vi "matrice_led.vi"() -> ()   [LabVIEW 2018]
panel:
  out "temp":u32
  in  "stop":bool
  in  "Meter":u32(knob) scale=0.0..10.0
  in  "Combo Box":string(combo)
  out "LED1 32":bool
  out "LED1 31":bool
  out "LED1 30":bool
  out "LED1 29":bool
  out "LED1 28":bool
  out "LED1 27":bool
  out "LED1 26":bool
  out "LED1 25":bool
  out "LED1 24":bool
  out "LED1 23":bool
  out "LED1 22":bool
  out "LED1 21":bool
  out "LED1 20":bool
  out "LED1 19":bool
  out "LED1 18":bool
  out "LED1 17":bool
  out "LED1 16":bool
  out "LED1 15":bool
  out "LED1 14":bool
  out "LED1 13":bool
  out "LED1 12":bool
  out "LED1 11":bool
  out "LED1 10":bool
  out "LED1 9":bool
  out "LED1 8":bool
  out "LED1 7":bool
  out "LED1 6":bool
  out "LED1 5":bool
  out "LED1 4":bool
  out "LED1 3":bool
  out "LED1 2":bool
  out "LED1":bool
  # "SIMULAREA UNOR EFECTE GRAFICE VARIATE CARE POT FI AFISATE PE MATRICEA VIRTUALA DE 8X4 LEDURI"
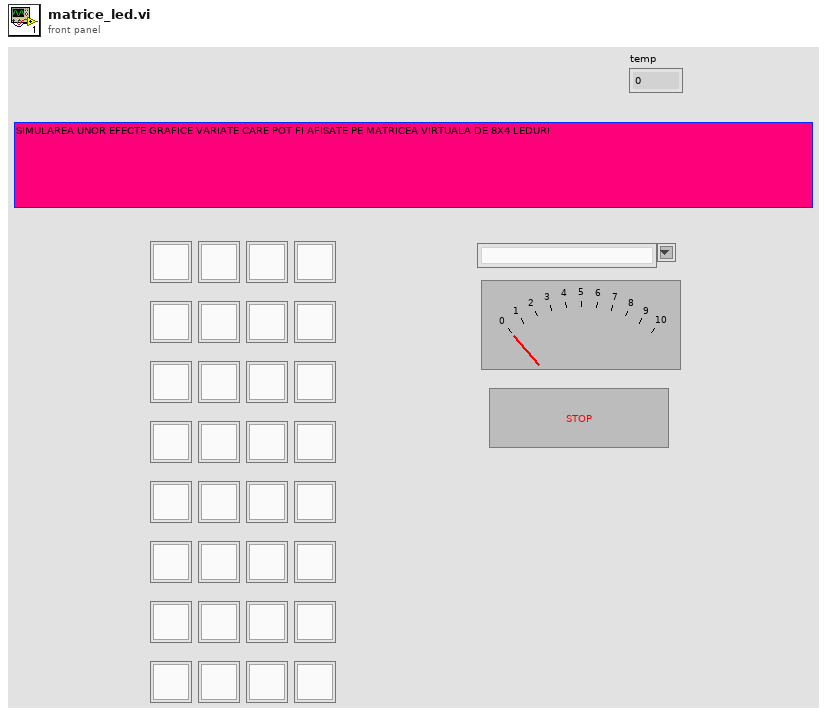
[diagram p1: front panel]
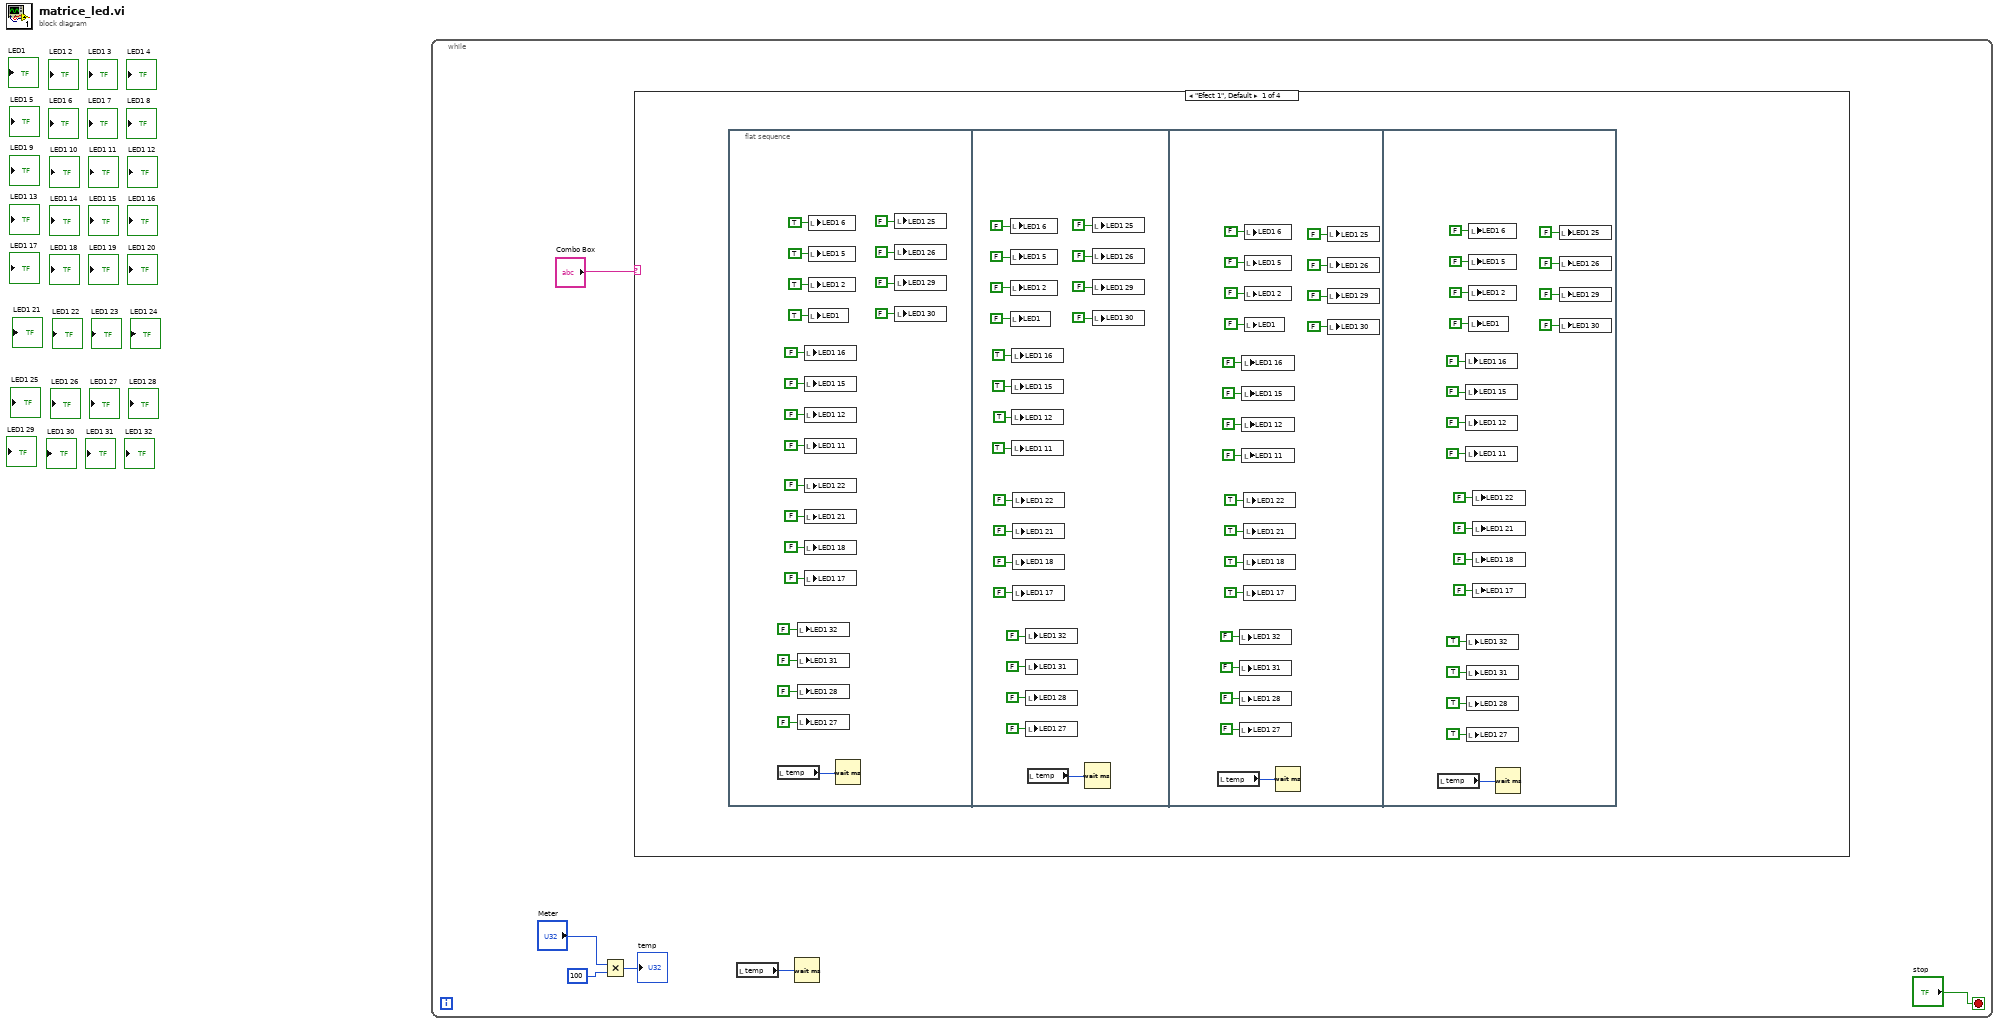
[diagram p0: block diagram]
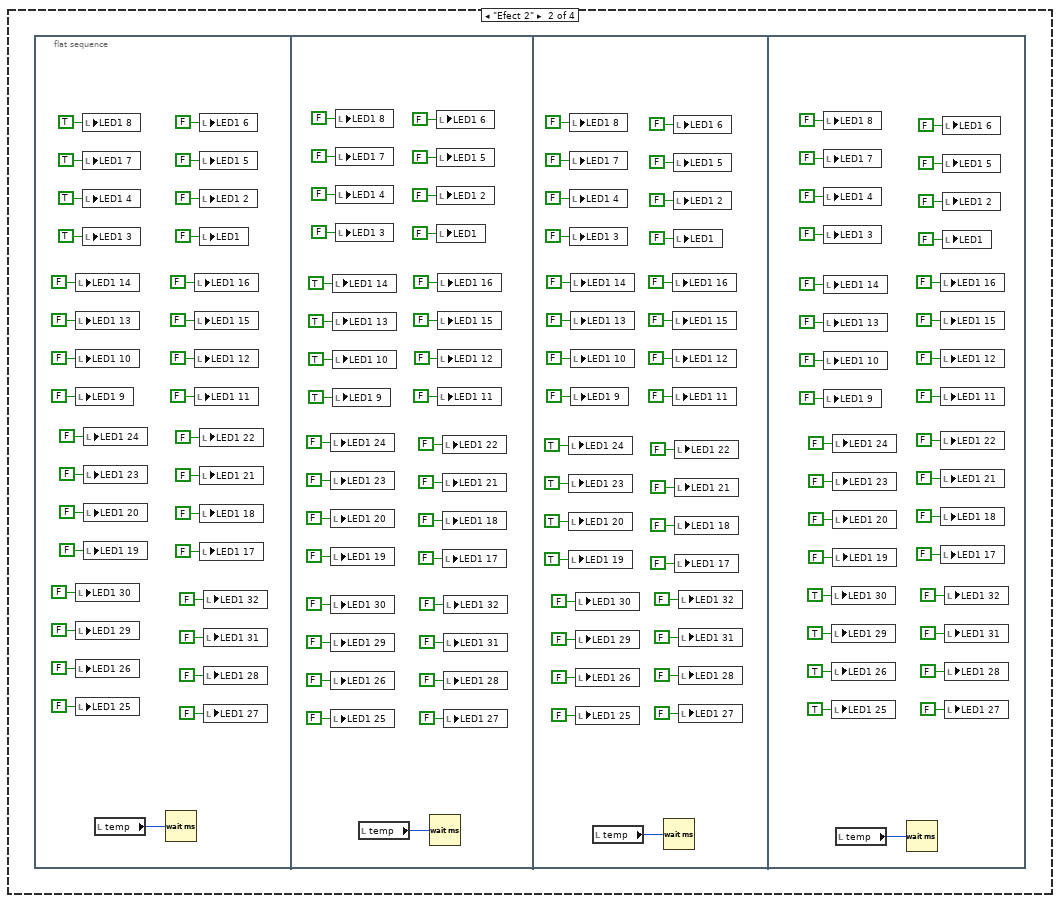
[diagram p2: hidden frame]
diagram:
  n1 = while {
    stop <- "stop" stop-if-true
    n2 = Multiply(x="Meter", y=u32 100) -> (x*y=→"temp":u32)
    n3 = case shown="\"Efect 1\", Default" "Combo Box" {
      frame "Efect 1", Default {
        n4 = flat-sequence {
          frame #0 {
            n5 = local read "temp"() -> (w27:u32)
            n6 = local write "LED1 32"(FALSE ("LED1 32")) -> ()
            n7 = local write "LED1 31"(FALSE ("LED1 31")) -> ()
            n8 = local write "LED1 28"(FALSE ("LED1 28")) -> ()
            n9 = local write "LED1 27"(FALSE ("LED1 27")) -> ()
            n10 = local write "LED1 16"(FALSE ("LED1 16")) -> ()
            n11 = local write "LED1 15"(FALSE ("LED1 15")) -> ()
            n12 = local write "LED1 12"(FALSE ("LED1 12")) -> ()
            n13 = local write "LED1 11"(FALSE ("LED1 11")) -> ()
            n14 = local write "LED1 22"(FALSE ("LED1 22")) -> ()
            n15 = local write "LED1 21"(FALSE ("LED1 21")) -> ()
            n16 = local write "LED1 18"(FALSE ("LED1 18")) -> ()
            n17 = local write "LED1 17"(FALSE ("LED1 17")) -> ()
            n18 = local write "LED1 6"(TRUE ("LED1 6")) -> ()
            n19 = local write "LED1 5"(TRUE ("LED1 5")) -> ()
            n20 = local write "LED1 2"(TRUE ("LED1 2")) -> ()
            n21 = local write "LED1"(TRUE ("LED1")) -> ()
            n22 = Wait (ms)(milliseconds to wait=w27) -> ()  [unwired: 1 out]
            n23 = local write "LED1 25"(FALSE ("LED1 25")) -> ()
            n24 = local write "LED1 26"(FALSE ("LED1 26")) -> ()
            n25 = local write "LED1 29"(FALSE ("LED1 29")) -> ()
            n26 = local write "LED1 30"(FALSE ("LED1 30")) -> ()
          }
          frame #1 {
            n27 = local write "LED1 6"(FALSE ("LED1 6")) -> ()
            n28 = local write "LED1 5"(FALSE ("LED1 5")) -> ()
            n29 = local write "LED1 2"(FALSE ("LED1 2")) -> ()
            n30 = local write "LED1"(FALSE ("LED1")) -> ()
            n31 = local write "LED1 16"(TRUE ("LED1 16")) -> ()
            n32 = local write "LED1 15"(TRUE ("LED1 15")) -> ()
            n33 = local write "LED1 12"(TRUE ("LED1 12")) -> ()
            n34 = local write "LED1 11"(TRUE ("LED1 11")) -> ()
            n35 = local write "LED1 22"(FALSE ("LED1 22")) -> ()
            n36 = local write "LED1 21"(FALSE ("LED1 21")) -> ()
            n37 = local write "LED1 18"(FALSE ("LED1 18")) -> ()
            n38 = local write "LED1 17"(FALSE ("LED1 17")) -> ()
            n39 = local write "LED1 32"(FALSE ("LED1 32")) -> ()
            n40 = local write "LED1 31"(FALSE ("LED1 31")) -> ()
            n41 = local write "LED1 28"(FALSE ("LED1 28")) -> ()
            n42 = local write "LED1 27"(FALSE ("LED1 27")) -> ()
            n43 = local read "temp"() -> (w48:u32)
            n44 = Wait (ms)(milliseconds to wait=w48) -> ()  [unwired: 1 out]
            n45 = local write "LED1 25"(FALSE ("LED1 25")) -> ()
            n46 = local write "LED1 26"(FALSE ("LED1 26")) -> ()
            n47 = local write "LED1 29"(FALSE ("LED1 29")) -> ()
            n48 = local write "LED1 30"(FALSE ("LED1 30")) -> ()
          }
          frame #2 {
            n49 = local read "temp"() -> (w69:u32)
            n50 = local write "LED1 32"(FALSE ("LED1 32")) -> ()
            n51 = local write "LED1 31"(FALSE ("LED1 31")) -> ()
            n52 = local write "LED1 28"(FALSE ("LED1 28")) -> ()
            n53 = local write "LED1 27"(FALSE ("LED1 27")) -> ()
            n54 = local write "LED1 16"(FALSE ("LED1 16")) -> ()
            n55 = local write "LED1 15"(FALSE ("LED1 15")) -> ()
            n56 = local write "LED1 12"(FALSE ("LED1 12")) -> ()
            n57 = local write "LED1 11"(FALSE ("LED1 11")) -> ()
            n58 = local write "LED1 22"(TRUE ("LED1 22")) -> ()
            n59 = local write "LED1 21"(TRUE ("LED1 21")) -> ()
            n60 = local write "LED1 18"(TRUE ("LED1 18")) -> ()
            n61 = local write "LED1 17"(TRUE ("LED1 17")) -> ()
            n62 = local write "LED1 6"(FALSE ("LED1 6")) -> ()
            n63 = local write "LED1 5"(FALSE ("LED1 5")) -> ()
            n64 = local write "LED1 2"(FALSE ("LED1 2")) -> ()
            n65 = local write "LED1"(FALSE ("LED1")) -> ()
            n66 = Wait (ms)(milliseconds to wait=w69) -> ()  [unwired: 1 out]
            n67 = local write "LED1 25"(FALSE ("LED1 25")) -> ()
            n68 = local write "LED1 26"(FALSE ("LED1 26")) -> ()
            n69 = local write "LED1 29"(FALSE ("LED1 29")) -> ()
            n70 = local write "LED1 30"(FALSE ("LED1 30")) -> ()
          }
          frame #3 {
            n71 = local read "temp"() -> (w90:u32)
            n72 = local write "LED1 16"(FALSE ("LED1 16")) -> ()
            n73 = local write "LED1 15"(FALSE ("LED1 15")) -> ()
            n74 = local write "LED1 12"(FALSE ("LED1 12")) -> ()
            n75 = local write "LED1 11"(FALSE ("LED1 11")) -> ()
            n76 = local write "LED1 32"(TRUE ("LED1 32")) -> ()
            n77 = local write "LED1 31"(TRUE ("LED1 31")) -> ()
            n78 = local write "LED1 28"(TRUE ("LED1 28")) -> ()
            n79 = local write "LED1 27"(TRUE ("LED1 27")) -> ()
            n80 = local write "LED1 6"(FALSE ("LED1 6")) -> ()
            n81 = local write "LED1 5"(FALSE ("LED1 5")) -> ()
            n82 = local write "LED1 2"(FALSE ("LED1 2")) -> ()
            n83 = local write "LED1"(FALSE ("LED1")) -> ()
            n84 = local write "LED1 22"(FALSE ("LED1 22")) -> ()
            n85 = local write "LED1 21"(FALSE ("LED1 21")) -> ()
            n86 = local write "LED1 18"(FALSE ("LED1 18")) -> ()
            n87 = local write "LED1 17"(FALSE ("LED1 17")) -> ()
            n88 = Wait (ms)(milliseconds to wait=w90) -> ()  [unwired: 1 out]
            n89 = local write "LED1 25"(FALSE ("LED1 25")) -> ()
            n90 = local write "LED1 26"(FALSE ("LED1 26")) -> ()
            n91 = local write "LED1 29"(FALSE ("LED1 29")) -> ()
            n92 = local write "LED1 30"(FALSE ("LED1 30")) -> ()
          }
        }
      }
      frame "Efect 2" {
        n93 = flat-sequence {
          frame #0 {
            n94 = local write "LED1 14"(FALSE ("LED1 14")) -> ()
            n95 = local write "LED1 13"(FALSE ("LED1 13")) -> ()
            n96 = local write "LED1 10"(FALSE ("LED1 10")) -> ()
            n97 = local write "LED1 9"(FALSE ("LED1 9")) -> ()
            n98 = local write "LED1 30"(FALSE ("LED1 30")) -> ()
            n99 = local write "LED1 29"(FALSE ("LED1 29")) -> ()
            n100 = local write "LED1 26"(FALSE ("LED1 26")) -> ()
            n101 = local write "LED1 25"(FALSE ("LED1 25")) -> ()
            n102 = local write "LED1 8"(TRUE ("LED1 8")) -> ()
            n103 = local write "LED1 7"(TRUE ("LED1 7")) -> ()
            n104 = local write "LED1 4"(TRUE ("LED1 4")) -> ()
            n105 = local write "LED1 3"(TRUE ("LED1 3")) -> ()
            n106 = local write "LED1 24"(FALSE ("LED1 24")) -> ()
            n107 = local write "LED1 23"(FALSE ("LED1 23")) -> ()
            n108 = local write "LED1 20"(FALSE ("LED1 20")) -> ()
            n109 = local write "LED1 19"(FALSE ("LED1 19")) -> ()
            n110 = local read "temp"() -> (w123:u32)
            n111 = Wait (ms)(milliseconds to wait=w123) -> ()  [unwired: 1 out]
            n112 = local write "LED1 16"(FALSE ("LED1 16")) -> ()
            n113 = local write "LED1 15"(FALSE ("LED1 15")) -> ()
            n114 = local write "LED1 12"(FALSE ("LED1 12")) -> ()
            n115 = local write "LED1 11"(FALSE ("LED1 11")) -> ()
            n116 = local write "LED1 6"(FALSE ("LED1 6")) -> ()
            n117 = local write "LED1 5"(FALSE ("LED1 5")) -> ()
            n118 = local write "LED1 2"(FALSE ("LED1 2")) -> ()
            n119 = local write "LED1"(FALSE ("LED1")) -> ()
            n120 = local write "LED1 22"(FALSE ("LED1 22")) -> ()
            n121 = local write "LED1 21"(FALSE ("LED1 21")) -> ()
            n122 = local write "LED1 18"(FALSE ("LED1 18")) -> ()
            n123 = local write "LED1 17"(FALSE ("LED1 17")) -> ()
            n124 = local write "LED1 32"(FALSE ("LED1 32")) -> ()
            n125 = local write "LED1 31"(FALSE ("LED1 31")) -> ()
            n126 = local write "LED1 28"(FALSE ("LED1 28")) -> ()
            n127 = local write "LED1 27"(FALSE ("LED1 27")) -> ()
          }
          frame #1 {
            n128 = local write "LED1 24"(FALSE ("LED1 24")) -> ()
            n129 = local write "LED1 23"(FALSE ("LED1 23")) -> ()
            n130 = local write "LED1 20"(FALSE ("LED1 20")) -> ()
            n131 = local write "LED1 19"(FALSE ("LED1 19")) -> ()
            n132 = local write "LED1 30"(FALSE ("LED1 30")) -> ()
            n133 = local write "LED1 29"(FALSE ("LED1 29")) -> ()
            n134 = local write "LED1 26"(FALSE ("LED1 26")) -> ()
            n135 = local write "LED1 25"(FALSE ("LED1 25")) -> ()
            n136 = local write "LED1 14"(TRUE ("LED1 14")) -> ()
            n137 = local write "LED1 13"(TRUE ("LED1 13")) -> ()
            n138 = local write "LED1 10"(TRUE ("LED1 10")) -> ()
            n139 = local write "LED1 9"(TRUE ("LED1 9")) -> ()
            n140 = local write "LED1 8"(FALSE ("LED1 8")) -> ()
            n141 = local write "LED1 7"(FALSE ("LED1 7")) -> ()
            n142 = local write "LED1 4"(FALSE ("LED1 4")) -> ()
            n143 = local write "LED1 3"(FALSE ("LED1 3")) -> ()
            n144 = local read "temp"() -> (w156:u32)
            n145 = Wait (ms)(milliseconds to wait=w156) -> ()  [unwired: 1 out]
            n146 = local write "LED1 6"(FALSE ("LED1 6")) -> ()
            n147 = local write "LED1 5"(FALSE ("LED1 5")) -> ()
            n148 = local write "LED1 2"(FALSE ("LED1 2")) -> ()
            n149 = local write "LED1"(FALSE ("LED1")) -> ()
            n150 = local write "LED1 16"(FALSE ("LED1 16")) -> ()
            n151 = local write "LED1 15"(FALSE ("LED1 15")) -> ()
            n152 = local write "LED1 12"(FALSE ("LED1 12")) -> ()
            n153 = local write "LED1 11"(FALSE ("LED1 11")) -> ()
            n154 = local write "LED1 22"(FALSE ("LED1 22")) -> ()
            n155 = local write "LED1 21"(FALSE ("LED1 21")) -> ()
            n156 = local write "LED1 18"(FALSE ("LED1 18")) -> ()
            n157 = local write "LED1 17"(FALSE ("LED1 17")) -> ()
            n158 = local write "LED1 32"(FALSE ("LED1 32")) -> ()
            n159 = local write "LED1 31"(FALSE ("LED1 31")) -> ()
            n160 = local write "LED1 28"(FALSE ("LED1 28")) -> ()
            n161 = local write "LED1 27"(FALSE ("LED1 27")) -> ()
          }
          frame #2 {
            n162 = local write "LED1 24"(TRUE ("LED1 24")) -> ()
            n163 = local write "LED1 23"(TRUE ("LED1 23")) -> ()
            n164 = local write "LED1 20"(TRUE ("LED1 20")) -> ()
            n165 = local write "LED1 19"(TRUE ("LED1 19")) -> ()
            n166 = local write "LED1 8"(FALSE ("LED1 8")) -> ()
            n167 = local write "LED1 7"(FALSE ("LED1 7")) -> ()
            n168 = local write "LED1 4"(FALSE ("LED1 4")) -> ()
            n169 = local write "LED1 3"(FALSE ("LED1 3")) -> ()
            n170 = local write "LED1 14"(FALSE ("LED1 14")) -> ()
            n171 = local write "LED1 13"(FALSE ("LED1 13")) -> ()
            n172 = local write "LED1 10"(FALSE ("LED1 10")) -> ()
            n173 = local write "LED1 9"(FALSE ("LED1 9")) -> ()
            n174 = local write "LED1 30"(FALSE ("LED1 30")) -> ()
            n175 = local write "LED1 29"(FALSE ("LED1 29")) -> ()
            n176 = local write "LED1 26"(FALSE ("LED1 26")) -> ()
            n177 = local write "LED1 25"(FALSE ("LED1 25")) -> ()
            n178 = local read "temp"() -> (w189:u32)
            n179 = Wait (ms)(milliseconds to wait=w189) -> ()  [unwired: 1 out]
            n180 = local write "LED1 16"(FALSE ("LED1 16")) -> ()
            n181 = local write "LED1 15"(FALSE ("LED1 15")) -> ()
            n182 = local write "LED1 12"(FALSE ("LED1 12")) -> ()
            n183 = local write "LED1 11"(FALSE ("LED1 11")) -> ()
            n184 = local write "LED1 6"(FALSE ("LED1 6")) -> ()
            n185 = local write "LED1 5"(FALSE ("LED1 5")) -> ()
            n186 = local write "LED1 2"(FALSE ("LED1 2")) -> ()
            n187 = local write "LED1"(FALSE ("LED1")) -> ()
            n188 = local write "LED1 22"(FALSE ("LED1 22")) -> ()
            n189 = local write "LED1 21"(FALSE ("LED1 21")) -> ()
            n190 = local write "LED1 18"(FALSE ("LED1 18")) -> ()
            n191 = local write "LED1 17"(FALSE ("LED1 17")) -> ()
            n192 = local write "LED1 32"(FALSE ("LED1 32")) -> ()
            n193 = local write "LED1 31"(FALSE ("LED1 31")) -> ()
            n194 = local write "LED1 28"(FALSE ("LED1 28")) -> ()
            n195 = local write "LED1 27"(FALSE ("LED1 27")) -> ()
          }
          frame #3 {
            n196 = local write "LED1 8"(FALSE ("LED1 8")) -> ()
            n197 = local write "LED1 7"(FALSE ("LED1 7")) -> ()
            n198 = local write "LED1 4"(FALSE ("LED1 4")) -> ()
            n199 = local write "LED1 3"(FALSE ("LED1 3")) -> ()
            n200 = local write "LED1 14"(FALSE ("LED1 14")) -> ()
            n201 = local write "LED1 13"(FALSE ("LED1 13")) -> ()
            n202 = local write "LED1 10"(FALSE ("LED1 10")) -> ()
            n203 = local write "LED1 9"(FALSE ("LED1 9")) -> ()
            n204 = local write "LED1 30"(TRUE ("LED1 30")) -> ()
            n205 = local write "LED1 29"(TRUE ("LED1 29")) -> ()
            n206 = local write "LED1 26"(TRUE ("LED1 26")) -> ()
            n207 = local write "LED1 25"(TRUE ("LED1 25")) -> ()
            n208 = local write "LED1 24"(FALSE ("LED1 24")) -> ()
            n209 = local write "LED1 23"(FALSE ("LED1 23")) -> ()
            n210 = local write "LED1 20"(FALSE ("LED1 20")) -> ()
            n211 = local write "LED1 19"(FALSE ("LED1 19")) -> ()
            n212 = local read "temp"() -> (w222:u32)
            n213 = Wait (ms)(milliseconds to wait=w222) -> ()  [unwired: 1 out]
            n214 = local write "LED1 16"(FALSE ("LED1 16")) -> ()
            n215 = local write "LED1 15"(FALSE ("LED1 15")) -> ()
            n216 = local write "LED1 12"(FALSE ("LED1 12")) -> ()
            n217 = local write "LED1 11"(FALSE ("LED1 11")) -> ()
            n218 = local write "LED1 22"(FALSE ("LED1 22")) -> ()
            n219 = local write "LED1 21"(FALSE ("LED1 21")) -> ()
            n220 = local write "LED1 18"(FALSE ("LED1 18")) -> ()
            n221 = local write "LED1 17"(FALSE ("LED1 17")) -> ()
            n222 = local write "LED1 6"(FALSE ("LED1 6")) -> ()
            n223 = local write "LED1 5"(FALSE ("LED1 5")) -> ()
            n224 = local write "LED1 2"(FALSE ("LED1 2")) -> ()
            n225 = local write "LED1"(FALSE ("LED1")) -> ()
            n226 = local write "LED1 32"(FALSE ("LED1 32")) -> ()
            n227 = local write "LED1 31"(FALSE ("LED1 31")) -> ()
            n228 = local write "LED1 28"(FALSE ("LED1 28")) -> ()
            n229 = local write "LED1 27"(FALSE ("LED1 27")) -> ()
          }
        }
      }
      frame "Efect 3" {
      }
      frame "Efect 4" {
      }
    }
    n230 = local read "temp"() -> (w1:u32)
    n231 = Wait (ms)(milliseconds to wait=w1) -> ()  [unwired: 1 out]
  }
